vi "automation_final_par_v2_new.vi"() -> ()   [LabVIEW 2013]
uses:
  <vilib>/DAQmx/write.llb/DAQmx Write (Digital Bool 1Line 1Point).vi
  <vilib>/DAQmx/create/channels.llb/DAQmx Create Channel (DO-Digital Output).vi
  <vilib>/DAQmx/miscellaneous.llb/DAQmx Fill In Error Info.vi
panel:
  in  "Start":bool
  in  "stop":bool
  in  "(half) steps":dbl
  in  "direction":bool
  out "dierection_task":refnum<k21> caption="Task (Ausgang)"
  out "steps_task":refnum<k21> caption="Task (Ausgang)"
  in  "Stepwidth":dbl(slide) min=0.0 max=3.0 step=1.0 scale=0.0..1.0 scale format="%#_3g"
  # "360° = 200 steps = 400 Halfsteps\n1 Step = 1,8°"
  # "stepper \nblk  _\nylw _3    \ngrn _3\n              m  m           \n              |  |  |\n           red wht blu\n\nstepper to driver\nblu  - wht\nred - gry\ngrn - vio\nblk - blu"
  # "clockwise"
  # "counterClockwise"
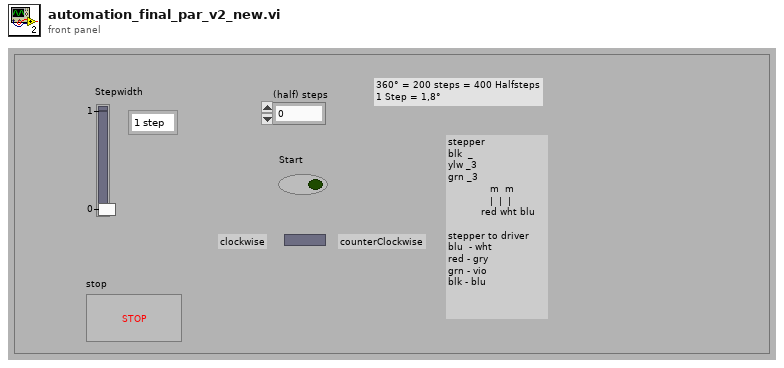
[diagram p1: front panel]
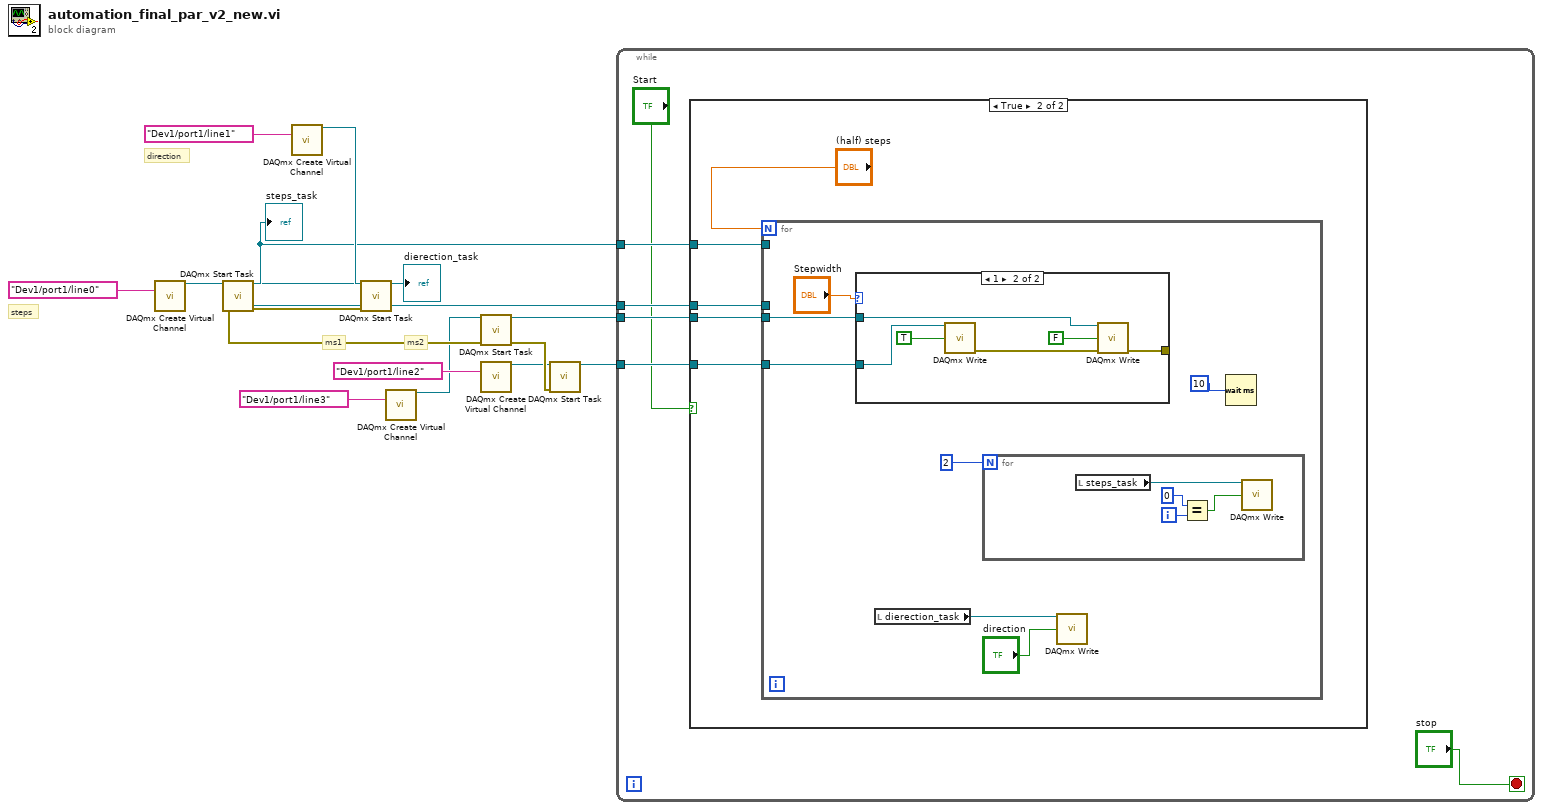
[diagram p0: block diagram]
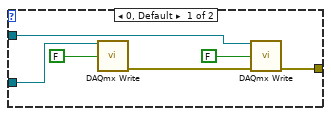
[diagram p3: hidden frame]
diagram:
  # "steps"
  # "direction"
  # "ms1"
  # "ms2"
  n1 = call-poly <vilib>:"DAQmx Create Virtual Channel.vi"("lines"=tag "Dev1/port1/line0") -> ("task out"=w8:refnum<k21>)  [unwired: 13 in, 1 out]
  n2 = call <vilib>:"DAQmx Start Task.vi"("task/channels in"=w8) -> ("task out"=w2:refnum<k21>, "error out"=w15:errorcluster)  [unwired: 13 in]
  "steps_task" <- w2
  n3 = call-poly <vilib>:"DAQmx Create Virtual Channel.vi"("lines"=tag "Dev1/port1/line1") -> ("task out"=w7:refnum<k21>)  [unwired: 13 in, 1 out]
  n4 = call <vilib>:"DAQmx Start Task.vi"("task/channels in"=w7, "error in"=w15) -> ("task out"=w1:refnum<k21>, "error out"=w9:errorcluster)  [unwired: 12 in]
  "dierection_task" <- w1
  n5 = call-poly <vilib>:"DAQmx Create Virtual Channel.vi"("lines"=tag "Dev1/port1/line3") -> ("task out"=w6:refnum<k21>)  [unwired: 13 in, 1 out]
  n6 = call <vilib>:"DAQmx Start Task.vi"("task/channels in"=w6, "error in"=w9) -> ("task out"=w3:refnum<k21>, "error out"=w10:errorcluster)  [unwired: 12 in]
  n7 = call-poly <vilib>:"DAQmx Create Virtual Channel.vi"("lines"=tag "Dev1/port1/line2") -> ("task out"=w5:refnum<k21>)  [unwired: 13 in, 1 out]
  n8 = call <vilib>:"DAQmx Start Task.vi"("task/channels in"=w5, "error in"=w10) -> ("task out"=w4:refnum<k21>)  [unwired: 12 in, 1 out]
  n9 = while {
    tunnel: w4 -> [w21]
    tunnel: w3 -> [w20]
    tunnel: w2 -> [w19]
    tunnel: w1 -> [w18]
    stop <- "stop" stop-if-true
    n10 = case shown="True" "Start" {
      tunnel: w21 -> [_ w26]
      tunnel: w20 -> [_ w25]
      tunnel: w19 -> [_ w24]
      tunnel: w18 -> [_ w23]
      frame False {
      }
      frame True {
        n11 = for {
          N: "(half) steps" -> [_]
          tunnel: w26 -> [w33]
          tunnel: w25 -> [w32]
          tunnel: w24 -> [_]
          tunnel: w23 -> [_]
          n12 = case shown="1" "Stepwidth" {
            tunnel: [w40 w46] -> _
            tunnel: w33 -> [w39 w45]
            tunnel: w32 -> [w38 w44]
            frame 0, Default {
              n13 = call-poly <vilib>:"DAQmx Write.vi"("task/channels in"=w39, "data"=FALSE) -> ("error out"=w41:errorcluster)  [unwired: 11 in, 2 out]
              n14 = call-poly <vilib>:"DAQmx Write.vi"("task/channels in"=w38, "data"=FALSE, "error in"=w41) -> ("error out"=w40:errorcluster)  [unwired: 10 in, 2 out]
            }
            frame 1 {
              n15 = call-poly <vilib>:"DAQmx Write.vi"("task/channels in"=w45, "data"=TRUE) -> ("error out"=w47:errorcluster)  [unwired: 11 in, 2 out]
              n16 = call-poly <vilib>:"DAQmx Write.vi"("task/channels in"=w44, "data"=FALSE, "error in"=w47) -> ("error out"=w46:errorcluster)  [unwired: 10 in, 2 out]
            }
          }
          n17 = local read "dierection_task"() -> (w29:refnum<k21>)
          n18 = for {
            N: 2 -> [_]
            i -> [w35]
            n19 = local read "steps_task"() -> (w37:refnum<k21>)
            n20 = Equal?(x=0, y=w35) -> (x = y?=w36:bool)
            n21 = call-poly <vilib>:"DAQmx Write.vi"("task/channels in"=w37, "data"=w36) -> ()  [unwired: 11 in, 3 out]
          }
          n22 = call-poly <vilib>:"DAQmx Write.vi"("task/channels in"=w29, "data"="direction") -> ()  [unwired: 11 in, 3 out]
          n23 = Wait (ms)(milliseconds to wait=10) -> ()  [unwired: 1 out]
        }
      }
    }
  }
